vi "XStage_Move.vi"(0 "Position":sgl, 1 "X_Wait":bool=TRUE) -> ()   [LabVIEW 2016]
uses:
  Utility/Global_Stage.vi
  Utility/Global Constants.vi
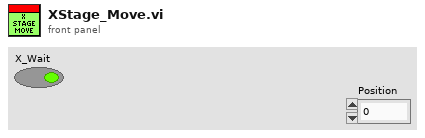
[diagram p1: front panel]
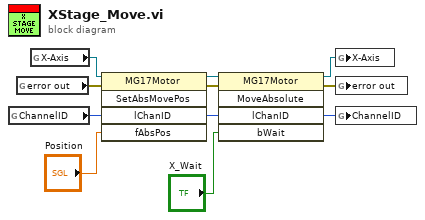
[diagram p0: block diagram]
diagram:
  n1 = global read "Global_Stage.vi" "ChannelID"() -> (w4:i32)
  n2 = global read "Global Constants.vi" "error out"() -> (w3:errorcluster)
  n3 = global read "Global_Stage.vi" "X-Axis"() -> (w6:refnum<k7>)
  n4 = invoke class="MG17Motor" method="SetAbsMovePos"(reference=w6, error in=w3, "lChanID"=w4, "fAbsPos"="Position") -> (reference out=w9:refnum<k7>, error out=w10:errorcluster, "lChanID"=w11:i32)  [unwired: 1 in, 2 out]
  n5 = invoke class="MG17Motor" method="MoveAbsolute"(reference=w9, error in=w10, "lChanID"=w11, "bWait"="X_Wait") -> (reference out=w5:refnum<k7>, error out=w2:errorcluster, "lChanID"=w1:i32)  [unwired: 1 in, 2 out]
  n6 = global write "Global_Stage.vi" "X-Axis"(w5) -> ()
  n7 = global write "Global Constants.vi" "error out"(w2) -> ()
  n8 = global write "Global_Stage.vi" "ChannelID"(w1) -> ()
